vi "Spinner Init.vi"(3 "Container State":T3, 4 "Previous State":variant, 5 "Previous Version":T2) -> (2 "Current State":T1)   [LabVIEW 2012, in "Spinner.xctl"]
uses:
  Spinner.xctl
  Spinner State.ctl
  <vilib>/_xctls/Container State.ctl
  <vilib>/_xctls/Version.ctl
  <vilib>/_xctls/XControlSupport.lvlib
panel:
  out "ignored error":errorcluster
  in  "Default Indicator State":T1
  in  "Default Control State":T1
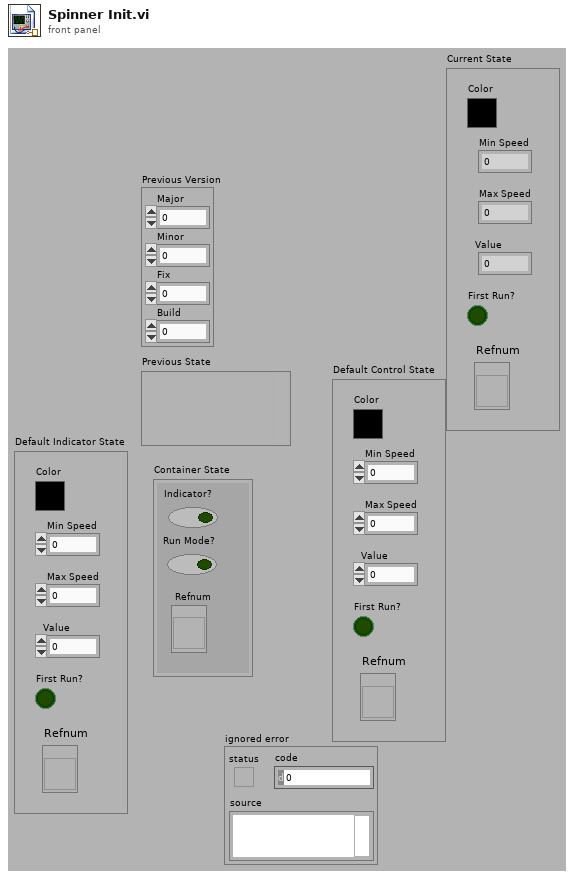
[diagram p1: front panel]
types:
  T1 = typedef "Spinner.xctl/Spinner State.ctl" = cluster{"Min Speed":dbl, "Color":u32, "Max Speed":dbl, "First Run?":bool, "Value":dbl, "Refnum":refnum<vi>}
  T2 = typedef "XControlSupport.lvlib/Version.ctl" = cluster{"Major":u16, "Minor":u16, "Fix":u16, "Build":u16}
  T3 = typedef "XControlSupport.lvlib/Container State.ctl" = cluster{"Indicator?":bool, "Run Mode?":bool, " Refnum":refnum<vi>}
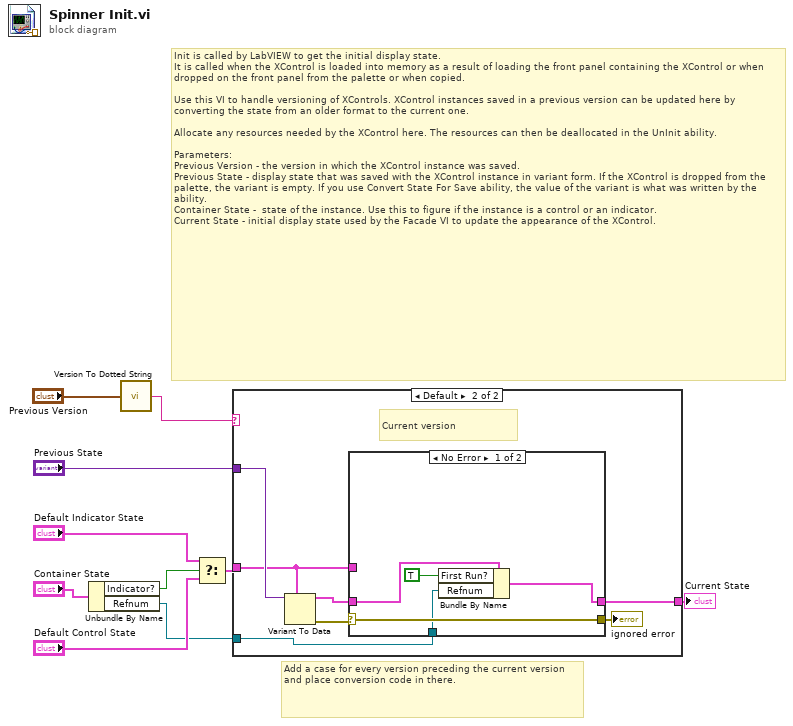
[diagram p0: block diagram]
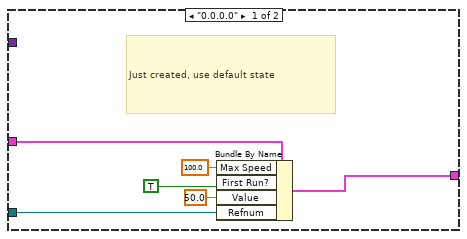
[diagram p2: hidden frame]
diagram:
  # "Add a case for every version preceding the current version and place conversion code in there."
  # "Init is called by LabVIEW to get the initial display state.\nIt is called when the XControl is loaded into memory as a result of loading the front panel containing the XControl or when dropped on the front panel from the palette or when copied.\n\nUse this VI to handle versioning of XControls. XControl instances saved in a previous version can be updated here by converting the state from an older format to the current one.\n\nAllocate any resources needed by the XControl here. The resources can then be deallocated in the UnInit ability.\n\nParameters:\nPrevious Version - the version in which the XControl instance was saved.\nPrevious State - display state that was saved with the XControl instance in variant form. If the XControl is dropped from the palette, the variant is empty. If you use Convert State For Save ability, the value of the variant is what was written by the ability. \nContainer State -  state of the instance. Use this to figure if the instance is a control or an indicator.\nCurrent State - initial display state used by the Facade VI to update the appearance of the XControl."
  n1 = Unbundle By Name("Container State") -> ("Indicator?"=w5:bool, "Refnum"=w1:refnum<vi>)
  n2 = call <vilib>:"Version To Dotted String.vi"("Version"="Previous Version") -> ("String Version"=w2:string)
  n3 = Select(t="Default Indicator State", s=w5, f="Default Control State") -> (s? t:f=w4:T1)
  n4 = case shown="Default" w2 {
    tunnel: "Previous State" -> [_ w23]
    tunnel: [w14 w19] -> w9
    tunnel: w4 -> [w16 w20]
    tunnel: w1 -> [w11 w17]
    frame "0.0.0.0" {
      # "Just created, use default state"
      n5 = Bundle By Name(cluster=w16, "Max Speed"=100.0, "First Run?"=TRUE, "Value"=50.0, "Refnum"=w11) -> (w14:T1)
    }
    frame Default {
      # "Current version"
      n6 = Variant To Data(type=w20, Variant=w23) -> (data=w21:T1, error out=w22:errorcluster)  [unwired: 1 in]
      n7 = case shown="No Error" w22 {
        selector: w22 -> [w28 w29]
        tunnel: w21 -> [w27 _]
        tunnel: [w26 w30] -> w19
        tunnel: w20 -> [_ w30]
        tunnel: [w28 w29] -> w18
        tunnel: w17 -> [w24 _]
        frame No Error {
          n8 = Bundle By Name(cluster=w27, "First Run?"=TRUE, "Refnum"=w24) -> (w26:T1)
        }
        frame Error {
          # "Error converting previously \nsaved state. Use default instead."
        }
      }
      "ignored error" <- w18
    }
  }
  "Current State" <- w9
